vi "Database Command Set Command Text.vi"(6 "CommandTimeout":i32, 7 "Prepared":bool, 8 "error in (no error)":errorcluster caption="错误输入（无错误）", 9 "CommandType":i32(ring)=1 items=["adCmdUnspecified"=-1, "adCmdUnknown"=8, "adCmdText"=1, "adCmdTable"=2, "adCmdStoredProc"=4, "adCmdFile"=256, "adCmdTableDirect"=512], 10 "CommandText":string, 11 "Database Command 输入":refnum<class "Database Command.lvclass"> caption="DNL_LabVIEW Object in") -> (0 "error out":errorcluster caption="错误输出", 3 "Database Command 输出":refnum<class "Database Command.lvclass"> caption="DNL_LabVIEW Object out")   [LabVIEW 2011, in "Database Command.lvclass"]
uses:
  Database Command.lvclass
  Database Command.lvclass/Database Command.ctl
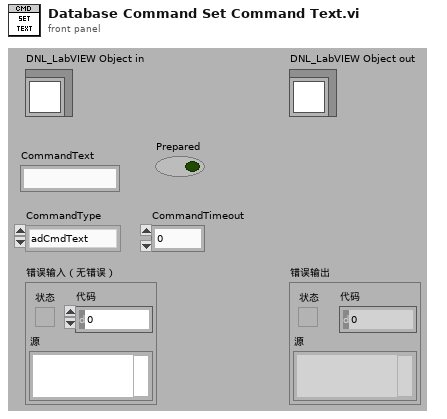
[diagram p1: front panel]
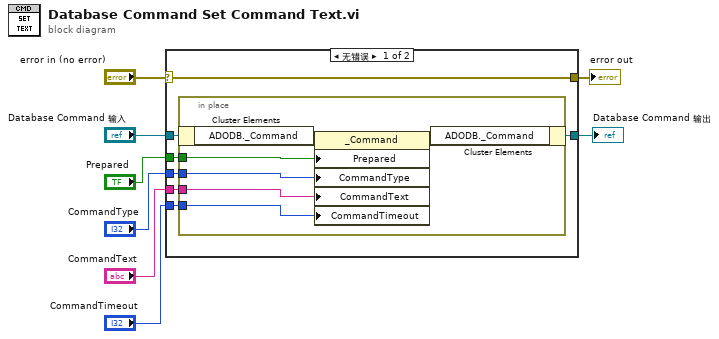
[diagram p0: block diagram]
diagram:
  n1 = case shown="无错误" "error in (no error)" {
    selector: "error in (no error)" -> [w15 w23]
    tunnel: [w15 w23] -> w7
    tunnel: [w13 w22] -> w5
    tunnel: "Database Command 输入" -> [w14 w22]
    tunnel: "Prepared" -> [w12 _]
    tunnel: "CommandType" -> [w11 _]
    tunnel: "CommandText" -> [w10 _]
    tunnel: "CommandTimeout" -> [w9 _]
    frame No Error {
      n2 = in-place {
        in-place-border: w12 -> [w19]
        in-place-border: w11 -> [w18]
        in-place-border: w10 -> [w17]
        in-place-border: w9 -> [w16]
        n3 = in-place-cluster #1(w14) -> ("ADODB._Command"=w21:refnum<k7>)
        n4 = property class="_Command"(reference=w21, "Prepared"=w19, "CommandType"=w18, "CommandText"=w17, "CommandTimeout"=w16) -> (reference out=w20:refnum<k7>)  [unwired: 1 in, 1 out]
        n5 = in-place-cluster #1("ADODB._Command"=w20) -> (w13:refnum<class "Database Command.lvclass">)
      }
    }
    frame Error {
    }
  }
  "error out" <- w7
  "Database Command 输出" <- w5
